vi "toStringArray.vi"(8 "error in (no error)":errorcluster, 11 "Delay in":refnum<class "Delay.lvclass">) -> (0 "error out":errorcluster, 2 "eventStringArray":string[](array[string]), 3 "Delay out":refnum<class "Delay.lvclass">)   [LabVIEW 2009, in "Tools.lvlib" / "Scripting.lvlib" / "Delay.lvclass"]
uses:
  Delay.lvclass
  ScriptEvent.lvclass
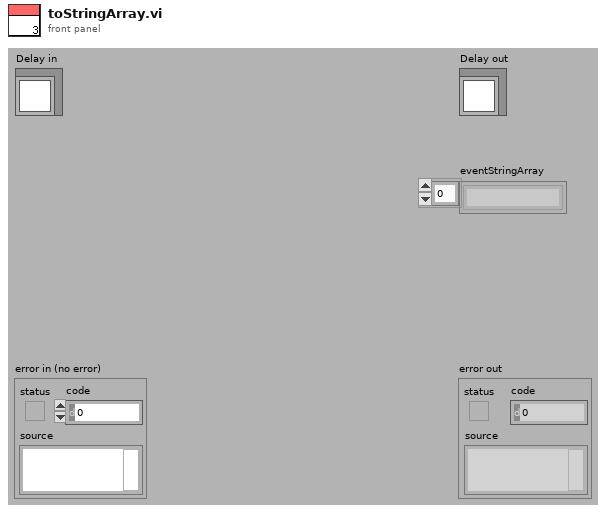
[diagram p1: front panel]
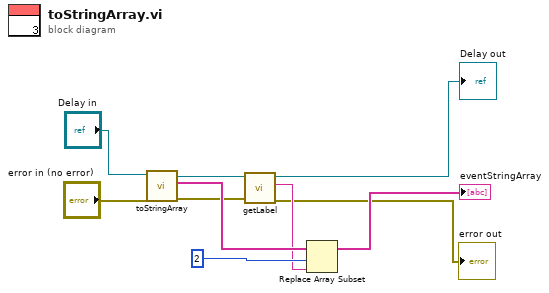
[diagram p0: block diagram]
diagram:
  n1 = call-parent "toStringArray.vi"("error in (no error)"="error in (no error)", "ScriptEvent in"="Delay in") -> ("error out"=w5:errorcluster, "eventStringArray"=w8:string[], "ScriptEvent out"=w6:refnum<class "Delay.lvclass">)  [unwired: 7 in]
  n2 = call "getLabel.vi"("error in (no error)"=w5, "Delay in"=w6) -> ("error out"=→"error out":errorcluster, "label"=w4:string, "Delay out"=→"Delay out":refnum<class "Delay.lvclass">)  [unwired: 7 in]
  n3 = Replace Array Subset(array=w8, new element=w4, index=2) -> (→"eventStringArray":string[])
